vi "Find Terminal by Label.vi"(10 "Terminal Label":string, 11 "VI":refnum<vi>) -> (2 "Found":bool, 3 "CtrlTerm Refnum":refnum<vi>)   [LabVIEW 2018, in "LVClassByRef.lvlib"]
uses:
  <resource>/Framework/Providers/LVClassByRef/LVClassByRef.lvlib
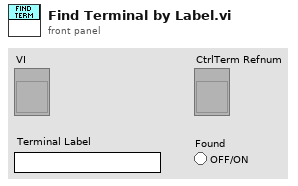
[diagram p1: front panel]
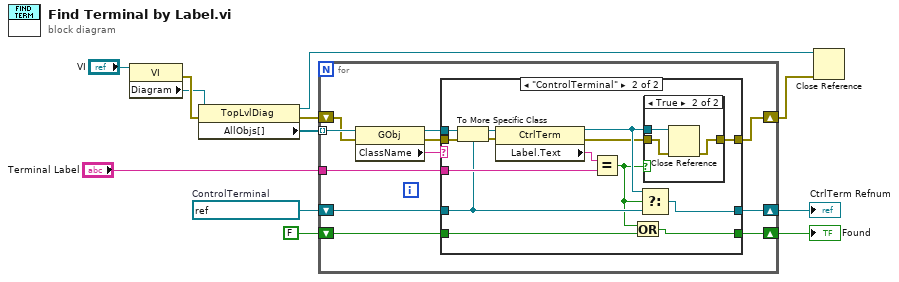
[diagram p0: block diagram]
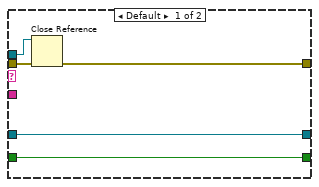
[diagram p2: hidden frame]
diagram:
  w4 = refnum<vi> refnum  # ControlTerminal
  n1 = property class="VI"(reference="VI") -> (error out=w12:errorcluster, "Diagram"=w11:refnum<vi>)  [unwired: 1 in, 1 out]
  n2 = property class="TopLvlDiag"(reference=w11, error in=w12) -> (reference out=w7:refnum<vi>, error out=w9:errorcluster, "AllObjs[]"=w10:refnum<vi>[])
  n3 = for {
    tunnel: w10 -> [w23] mode=indexing
    shift-right: [w18] -> w8
    shift-left: w9 -> [w20]
    tunnel: "Terminal Label" -> [w17]
    shift-right: [w15] -> w3
    shift-left: w4 -> [w16]
    shift-right: [w13] -> w1
    shift-left: FALSE -> [w14]
    n4 = property class="GObj"(reference=w23, error in=w20) -> (reference out=w21:refnum<vi>, error out=w19:errorcluster, "ClassName"=w22:string)
    n5 = case shown="\"ControlTerminal\"" w22 {
      tunnel: w21 -> [w27 w42]
      tunnel: w19 -> [w28 w40]
      tunnel: [w26 w34] -> w18
      tunnel: w17 -> [_ w37]
      tunnel: w16 -> [w25 w32]
      tunnel: [w25 w33] -> w15
      tunnel: w14 -> [w24 w30]
      tunnel: [w24 w29] -> w13
      frame Default {
        n6 = Close Reference(reference=w27, error in (no error)=w28) -> (error out=w26:errorcluster)
      }
      frame "ControlTerminal" {
        n7 = To More Specific Class(target class=w32, reference=w42, error in=w40) -> (specific class reference=w41:refnum<vi>, error out=w39:errorcluster)
        n8 = property class="CtrlTerm"(reference=w41, error in=w39) -> (reference out=w36:refnum<vi>, error out=w35:errorcluster, "Label.Text"=w38:string)
        n9 = Equal?(x=w38, y=w37) -> (x = y?=w31:bool)
        n10 = Or(x=w31, y=w30) -> (x .or. y?=w29:bool)
        n11 = Select(t=w36, s=w31, f=w32) -> (s? t:f=w33:refnum<vi>)
        n12 = case shown="True" w31 {
          tunnel: w36 -> [_ w46]
          tunnel: w35 -> [w43 w45]
          tunnel: [w43 w44] -> w34
          frame False {
          }
          frame True {
            n13 = Close Reference(reference=w46, error in (no error)=w45) -> (error out=w44:errorcluster)
          }
        }
      }
    }
  }
  "CtrlTerm Refnum" <- w3
  "Found" <- w1
  n14 = Close Reference(reference=w7, error in (no error)=w8) -> ()  [unwired: 1 out]
